vi "Lookup Format String.vi"(8 "error in":errorcluster, 9 "element":T2=enum."Boolean", 10 "Type Formatting":T1) -> (0 "error out":errorcluster, 1 "found?":bool, 2 "Format String":string, 4 "custom?":bool)   [LabVIEW 2011]
uses:
  Type Defs/Formatting Data Type -- Enum.ctl
  Options API/Private/EasyXML Options - Type Formatting Cluster.ctl
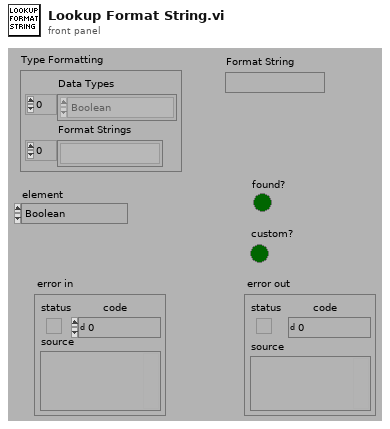
[diagram p1: front panel]
types:
  T1 = typedef "EasyXML Options - Type Formatting Cluster.ctl" = cluster{"Data Types":T2[], "Format Strings":string[]}
  T2 = typedef "Formatting Data Type -- Enum.ctl" = enum16{"<unknown>", "Cluster", "Array", "String", "Path", "Boolean", "Time Stamp", "Enum", "Numeric - EXT", "Numeric - DBL", "Numeric - SGL", "Numeric - I64", "Numeric - I32", "Numeric - I16", "Numeric - I8", "Numeric - U64", "Numeric - U32", "Numeric - U16", "Numeric - U8", "Numeric - CXT", "Numeric - CDB", "Numeric - CSG", "VISA Resource"}
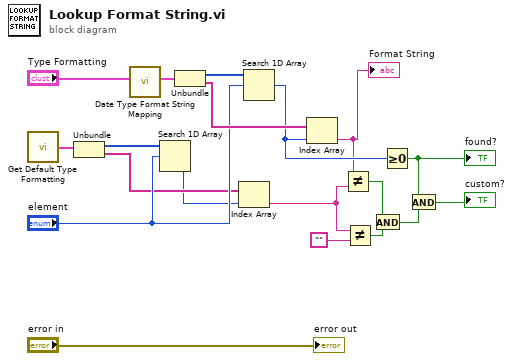
[diagram p0: block diagram]
diagram:
  n1 = call "Get Default Type Formatting.vi"() -> ("Default Type Formatting"=w2:T1)
  n2 = Unbundle(w2) -> ("Data Types"=w14:T2[], "Format Strings"=w12:string[])
  n3 = call "Date Type Format String Mapping.vi"("Type Formatting"="Type Formatting") -> ("Type Formatting populated"=w17:T1)  [unwired: 10 in]
  n4 = Search 1D Array(1D array=w14, element="element") -> (index of element=w11:i32)  [unwired: 1 in]
  n5 = Unbundle(w17) -> ("Data Types"=w18:T2[], "Format Strings"=w19:string[])
  n6 = Index Array(array=w12, index=w11) -> (element=w6:string)
  n7 = Search 1D Array(1D array=w18, element="element") -> (index of element=w15:i32)  [unwired: 1 in]
  n8 = Index Array(array=w19, index=w15) -> (element=w10:string)
  "Format String" <- w10
  n9 = Not Equal?(x=w10, y=w6) -> (x != y?=w7:bool)
  n10 = Not Equal?(x=w6, y="") -> (x != y?=w4:bool)
  n11 = And(x=w7, y=w4) -> (x .and. y?=w3:bool)
  n12 = Greater Or Equal To 0?(x=w15) -> (x >= 0?=w9:bool)
  "found?" <- w9
  n13 = And(x=w9, y=w3) -> (x .and. y?=→"custom?":bool)
  "error out" <- "error in"
